vi "Drag Edges.vi"(0 "FSM in":refnum<class "FSM.Graph.lvclass">, 9 "delta":cluster{"X":dbl, "Y":dbl}, 11 "error in (no error)":errorcluster) -> (4 "FSM out":refnum<class "FSM.Graph.lvclass">, 15 "error out":errorcluster)   [LabVIEW 2015, in "FSM.Graph.lvclass"]
uses:
  FSM.Graph.lvclass
  FSM.Graph.lvclass/FSM.Graph.ctl
  FSM.Edge/FSM.Edge.lvclass
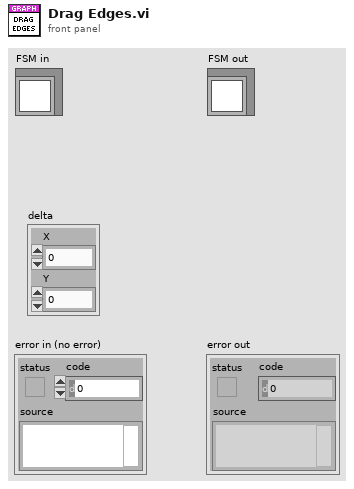
[diagram p1: front panel]
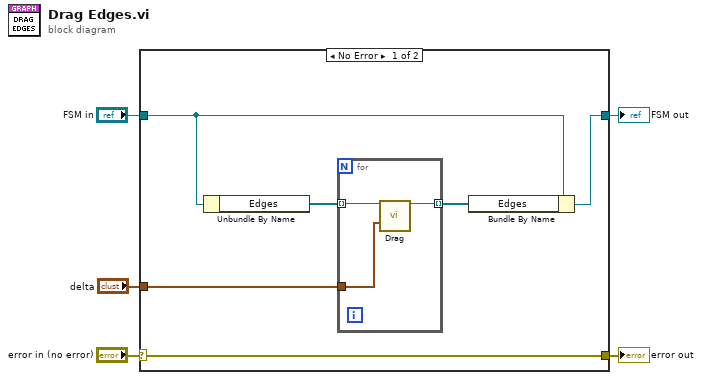
[diagram p0: block diagram]
diagram:
  n1 = case shown="No Error" "error in (no error)" {
    selector: "error in (no error)" -> [w11 w16]
    tunnel: [w11 w16] -> w4
    tunnel: [w8 w15] -> w2
    tunnel: "FSM in" -> [w10 w15]
    tunnel: "delta" -> [w6 _]
    frame No Error {
      n2 = Unbundle By Name(w10) -> ("Edges"=w9:refnum<class "FSM.Edge.lvclass">[])
      n3 = for {
        tunnel: w6 -> [w12]
        tunnel: w9 -> [w14] mode=indexing
        tunnel: [w13] -> w7 mode=indexing
        n4 = call "Drag.vi"("FSM.Edge in"=w14, "delta"=w12) -> ("FSM.Edge out"=w13:refnum<class "FSM.Edge.lvclass">)  [unwired: 13 in]
      }
      n5 = Bundle By Name(cluster=w10, "Edges"=w7) -> (w8:refnum<class "FSM.Graph.lvclass">)
    }
    frame Error {
    }
  }
  "error out" <- w4
  "FSM out" <- w2
